vi "Collector.vi"   [LabVIEW 2012]
uses:
  StateMachineEnum.ctl
  <vilib>/Rock Robotics/WPI/Relay/WPI_RelayValue.ctl
  Robot Global Data.vi
types:
  T1 = typedef "StateMachineEnum.ctl" = enum16{"Init", "Idle", "Start", "Do", "Stop"}
  T2 = typedef "WPI_RelayValue.ctl" = enum16{"Off", "On", "Forward", "Reverse"}
  T3 = typedef "WPI_RelayDevRef.ctl" = cluster{"DevStatus":errorcluster, "Relay Channel":T4, "Digital Module":T5, "Relay Direction":T6}
  T4 = typedef "FPGA_DIORelayChannel.ctl" = enum8{"Relay 1", "Relay 2", "Relay 3", "Relay 4", "Relay 5", "Relay 6", "Relay 7", "Relay 8", "Invalid"}
  T5 = typedef "FPGA_TypedefDigitalModule.ctl" = enum16{"Digital Module 1", "Digital Module 2"}
  T6 = typedef "WPI_RelayDirection.ctl" = enum16{"Both directions", "Forward only", "Reverse only"}
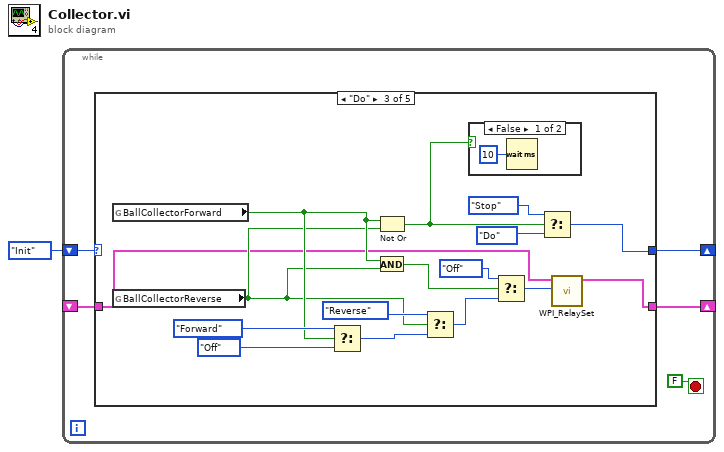
[diagram p0: block diagram]
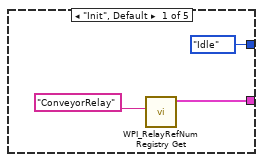
[diagram p2: hidden frame]
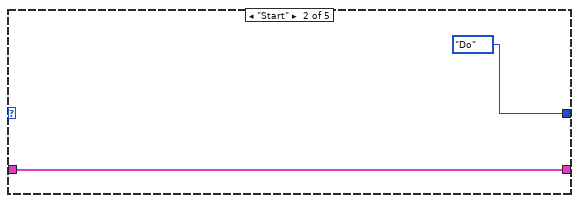
[diagram p3: hidden frame]
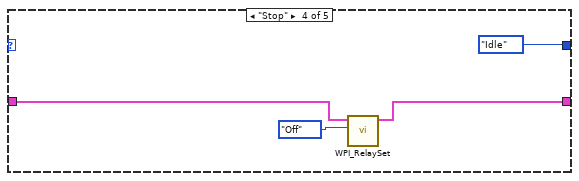
[diagram p5: hidden frame]
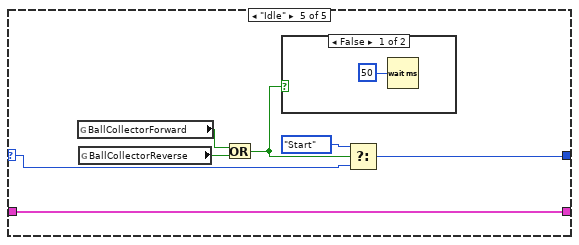
[diagram p6: hidden frame]
diagram:
  n1 = while {
    shift-right: [w5] -> _
    shift-left: StateMachineEnum."Init" ("State") -> [w6]
    shift-right: [w4] -> _
    shift-left: _ -> [w2]
    stop <- FALSE stop-if-true
    n2 = case shown="\"Do\"" w6 {
      selector: w6 -> [_ _ _ _ w36]
      tunnel: [StateMachineEnum."Idle" ("State") StateMachineEnum."Do" ("State") w15 StateMachineEnum."Idle" ("State") w34] -> w5
      tunnel: [w8 w10 w14 w30 w33] -> w4
      tunnel: w2 -> [_ w10 w13 w31 w33]
      frame "Init", Default {
        n3 = call <vilib>:"WPI_RelayRefNum Registry Get.vi"("refnum name"="ConveyorRelay") -> ("RelayDevRef"=w8:T3)  [unwired: 9 in, 1 out]
      }
      frame "Start" {
      }
      frame "Do" {
        n4 = global read "Robot Global Data.vi" "BallCollectorForward"() -> (w20:bool)
        n5 = global read "Robot Global Data.vi" "BallCollectorReverse"() -> (w16:bool)
        n6 = Select(t=WPI_RelayValue."Forward" ("RelayValue"), s=w20, f=WPI_RelayValue."Off" ("RelayValue")) -> (s? t:f=w23:T2)
        n7 = Not Or(1:w16, 2:w20) -> (0:w12:bool)
        n8 = And(x=w20, y=w16) -> (x .and. y?=w19:bool)
        n9 = Select(t=WPI_RelayValue."Reverse" ("RelayValue"), s=w16, f=w23) -> (s? t:f=w18:T2)
        n10 = case shown="False" w12 {
          frame False {
            n11 = Wait (ms)(milliseconds to wait=u32 10) -> ()  [unwired: 1 out]
          }
          frame True {
          }
        }
        n12 = Select(t=WPI_RelayValue."Off" ("RelayValue"), s=w19, f=w18) -> (s? t:f=w21:T2)
        n13 = Select(t=StateMachineEnum."Stop" ("State"), s=w12, f=StateMachineEnum."Do" ("State")) -> (s? t:f=w15:T1)
        n14 = call <vilib>:"WPI_RelaySet.vi"("RelayValue"=w21, "RelayDevRef"=w13) -> ("RelayDevRef"=w14:T3)  [unwired: 8 in, 1 out]
      }
      frame "Stop" {
        n15 = call <vilib>:"WPI_RelaySet.vi"("RelayValue"=WPI_RelayValue."Off", "RelayDevRef"=w31) -> ("RelayDevRef"=w30:T3)  [unwired: 8 in, 1 out]
      }
      frame "Idle" {
        n16 = global read "Robot Global Data.vi" "BallCollectorForward"() -> (w39:bool)
        n17 = global read "Robot Global Data.vi" "BallCollectorReverse"() -> (w38:bool)
        n18 = Or(x=w39, y=w38) -> (x .or. y?=w37:bool)
        n19 = case shown="False" w37 {
          frame False {
            n20 = Wait (ms)(milliseconds to wait=u32 50) -> ()  [unwired: 1 out]
          }
          frame True {
          }
        }
        n21 = Select(t=StateMachineEnum."Start" ("State"), s=w37, f=w36) -> (s? t:f=w34:T1)
      }
    }
  }
